vi "Iterate.vi"(11 "Grid.lvclass 2":refnum<class "Grid.lvclass">) -> (3 "Grid.lvclass":refnum<class "Grid.lvclass">)   [LabVIEW 2016, in "Grid.lvclass"]
uses:
  Grid.lvclass
  Pixel/Pixel.lvclass
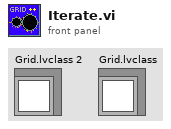
[diagram p1: front panel]
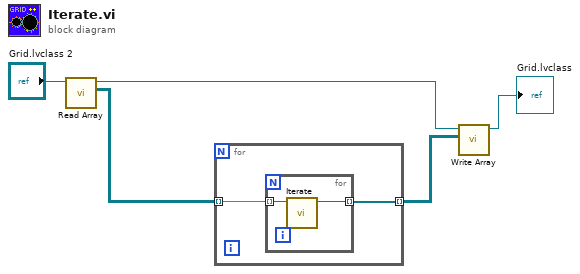
[diagram p0: block diagram]
diagram:
  n1 = call-dynamic "Read Array.vi"("Grid in"="Grid.lvclass 2") -> ("Grid"=w5:refnum<class "Pixel.lvclass">[][], "Grid out"=w4:refnum<class "Grid.lvclass">)  [unwired: 8 in, 1 out]
  n2 = for {
    tunnel: w5 -> [w7] mode=indexing
    tunnel: [w6] -> w3 mode=indexing
    n3 = for {
      tunnel: w7 -> [w9] mode=indexing
      tunnel: [w8] -> w6 mode=indexing
      n4 = call "Iterate.vi"("Pixel In"=w9) -> ("Pixel Outs"=w8:refnum<class "Pixel.lvclass">)  [unwired: 9 in, 1 out]
    }
  }
  n5 = call-dynamic "Write Array.vi"("Grid"=w3, "Grid in"=w4) -> ("Grid out"=→"Grid.lvclass":refnum<class "Grid.lvclass">)  [unwired: 8 in, 1 out]
